vi "set_params.vi"(8 "error in (no error)":errorcluster caption="entrée d'erreur (pas d'erreur)", 11 "TSNE.lvclass 2":refnum<class "TSNE.lvclass">) -> (0 "error out":errorcluster caption="sortie d'erreur", 3 "TSNE.lvclass":refnum<class "TSNE.lvclass">)   [LabVIEW 2020, in "TSNE.lvclass"]
uses:
  TSNE.lvclass
  TSNE.lvclass/TSNE.ctl
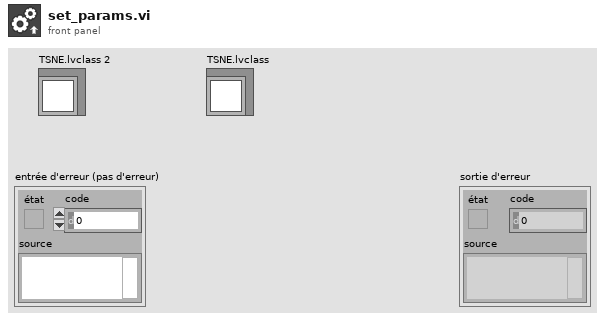
[diagram p1: front panel]
types:
  T1 = typedef "tsne_params.ctl" = cluster{"n_components":dbl, "perplexity":dbl, "early_exaggeration":dbl, "learning_rate":dbl, "n_iter":dbl, "n_iter_without_progress":dbl, "min_grad_norm":dbl, "metric":cluster{"metric_type":string, "metric_function":string}, "init":cluster{"init_type":string, "init_list":dbl[][]}, "verbose":dbl, "random_state":dbl, "method":string, "angle":dbl, "n_jobs":dbl}
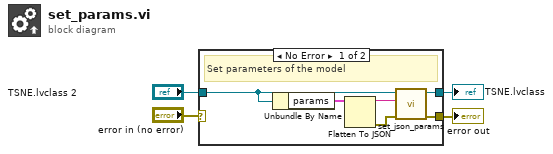
[diagram p0: block diagram]
diagram:
  n1 = case shown="No Error" "error in (no error)" {
    selector: "error in (no error)" -> [_ w12]
    tunnel: [w7 w12] -> w3
    tunnel: [w8 w11] -> w1
    tunnel: "TSNE.lvclass 2" -> [w5 w11]
    frame No Error {
      # "Set parameters of the model"
      n2 = Unbundle By Name(w5) -> ("params"=w10:T1)
      n3 = Flatten To JSON(anything=w10) -> (JSON string=w9:string, 11:w6:errorcluster)  [unwired: 2 in]
      n4 = call-dynamic "set_json_params.vi"("error in (no error)"=w6, "params"=w9, "Model en entrée"=w5) -> ("error out"=w7:errorcluster, "Model en sortie"=w8:refnum<class "TSNE.lvclass">)  [unwired: 7 in]
    }
    frame Error {
    }
  }
  "error out" <- w3
  "TSNE.lvclass" <- w1
